vi "CODMn测量数据储存.vi"   [LabVIEW 2016, in "斯坦道CODMn新电路板.lvlib"]
uses:
  <vilib>/ptbypt/NI_PtbyPt.lvlib
types:
  T1 = cluster{"时间标识":timestamp, "监测值":sgl, "单位":u16, "数据标识":string, "因子编码":u32, "标样参考值":sgl, "A":sgl, "B":sgl, "K":sgl, "终点滴定数":sgl, "环境温度":sgl, "环境湿度":sgl, "量程":sgl, "加热实时温度":sgl, "X0":sgl, "X^2":sgl, "X":sgl, "B 2":sgl, "跨度值":sgl, "光值1":sgl, "光值2":sgl, "光值3":sgl, "光值4":sgl, "光值5":sgl, "光值6":sgl, "光值7":sgl, "光值8":sgl}
  T2 = enum16{"维护数据", "水样测试", "标样核查", "零点核查", "跨度核查", "空白测试", "平行样测试", "加标回收", "空白校准", "标样校准", "初始化（清洗）"}
  T3 = cluster{"系统时间":timestamp, "工作状态":u16, "测量模式":enum16{"待机", "连续模式", "周期模式", "定点模式", "受控模式", "手动模式"}, "告警代码":u16, "故障代码":u16, "日志代码":u16, "软件版本":u16, "A":sgl, "B":sgl, "K":sgl, "当前滴定数":sgl, "T":sgl, "H":sgl, "id":u16, "flowid":u16, "量程":u16, "加热实时温度":sgl, "当前ORP值":sgl, "运行时间":sgl, "当前步骤剩余时间":sgl, "结束滴定数":sgl, "注射泵保温温度":sgl, "匹配滴定数X0":u16, "X^2":sgl, "X":sgl, "B 2":sgl, "光值1":sgl, "光值2":sgl, "光值3":sgl, "光值4":sgl, "光值5":sgl, "光值6":sgl, "光值7":sgl, "光值8":sgl}
  T4 = enum16{"水样测试", "标样核查", "跨度核查", "零点核查", "空白测试", "平行样测试", "加标回收", "空白校准", "标样校准"}[]
  T5 = cluster{"运行模式":enum16{"维护模式", "常规模式", "应急模式", "质控模式", "性能测试"}, "质控频次":enum16{"关闭", "每天", "星期一", "星期二", "星期三", "星期四", "星期五", "星期六", "星期日"}, "空白核查时间":u16, "跨度核查时间":u16, "测量间隔":u16}
  T6 = cluster{"因子编码":u32, "单位":u16, "标样参考值":sgl, "水样数据时间":timestamp, "水样实测值":sgl, "水样数据标识":string, "标样数据时间":timestamp, "标样实测值":sgl, "标样数据标识":string, "空白数据时间":timestamp, "空白实测值":sgl, "空白数据标识":string, "零点核查数据时间":timestamp, "零点核查实测值":sgl, "零点核查数据标识":string, "跨度核查数据时间":timestamp, "跨度核查实测值":sgl, "跨度核查数据标识":string, "加标回收数据时间":timestamp, "加标回收实测值":sgl, "加标回收数据标识":string, "平行样数据时间":timestamp, "平行样实测值":sgl, "平行样数据标识":string, "F0":sgl, "F1":sgl, "F2":sgl, "F3":sgl, "F4":sgl, "F5":sgl, "F6":sgl, "F7":sgl, "温度":sgl, "湿度":sgl, "X值":sgl, "fidrange":u16}
  T7 = cluster{"跨度值":dbl, "零点标准液浓度":dbl, "跨度标准液浓度":dbl, "标准液标准浓度":dbl, "零点标准液偏差":dbl, "跨度标准液偏差":dbl, "标准液标准偏差":dbl}
  T8 = cluster{"公式":cluster{"X^2":dbl, "X":dbl, "B":dbl}, "校准":cluster{"校准？":bool, "校准点1-5":u16, "校准浓度":dbl}}
  T9 = cluster{"测量量程":sgl, "测量检出限":sgl, "测量精度":sgl, "测量间隔":sgl, "消解温度":sgl, "消解时长":sgl, "三项式系数":sgl, "二次多项式系数":sgl, "曲线斜率":sgl, "曲线截距":sgl, "线性相关系数":sgl, "空白校准时间":timestamp, "标样校准时间":timestamp, "测量信号值":sgl, "稀释倍数":sgl, "量程系数":sgl}
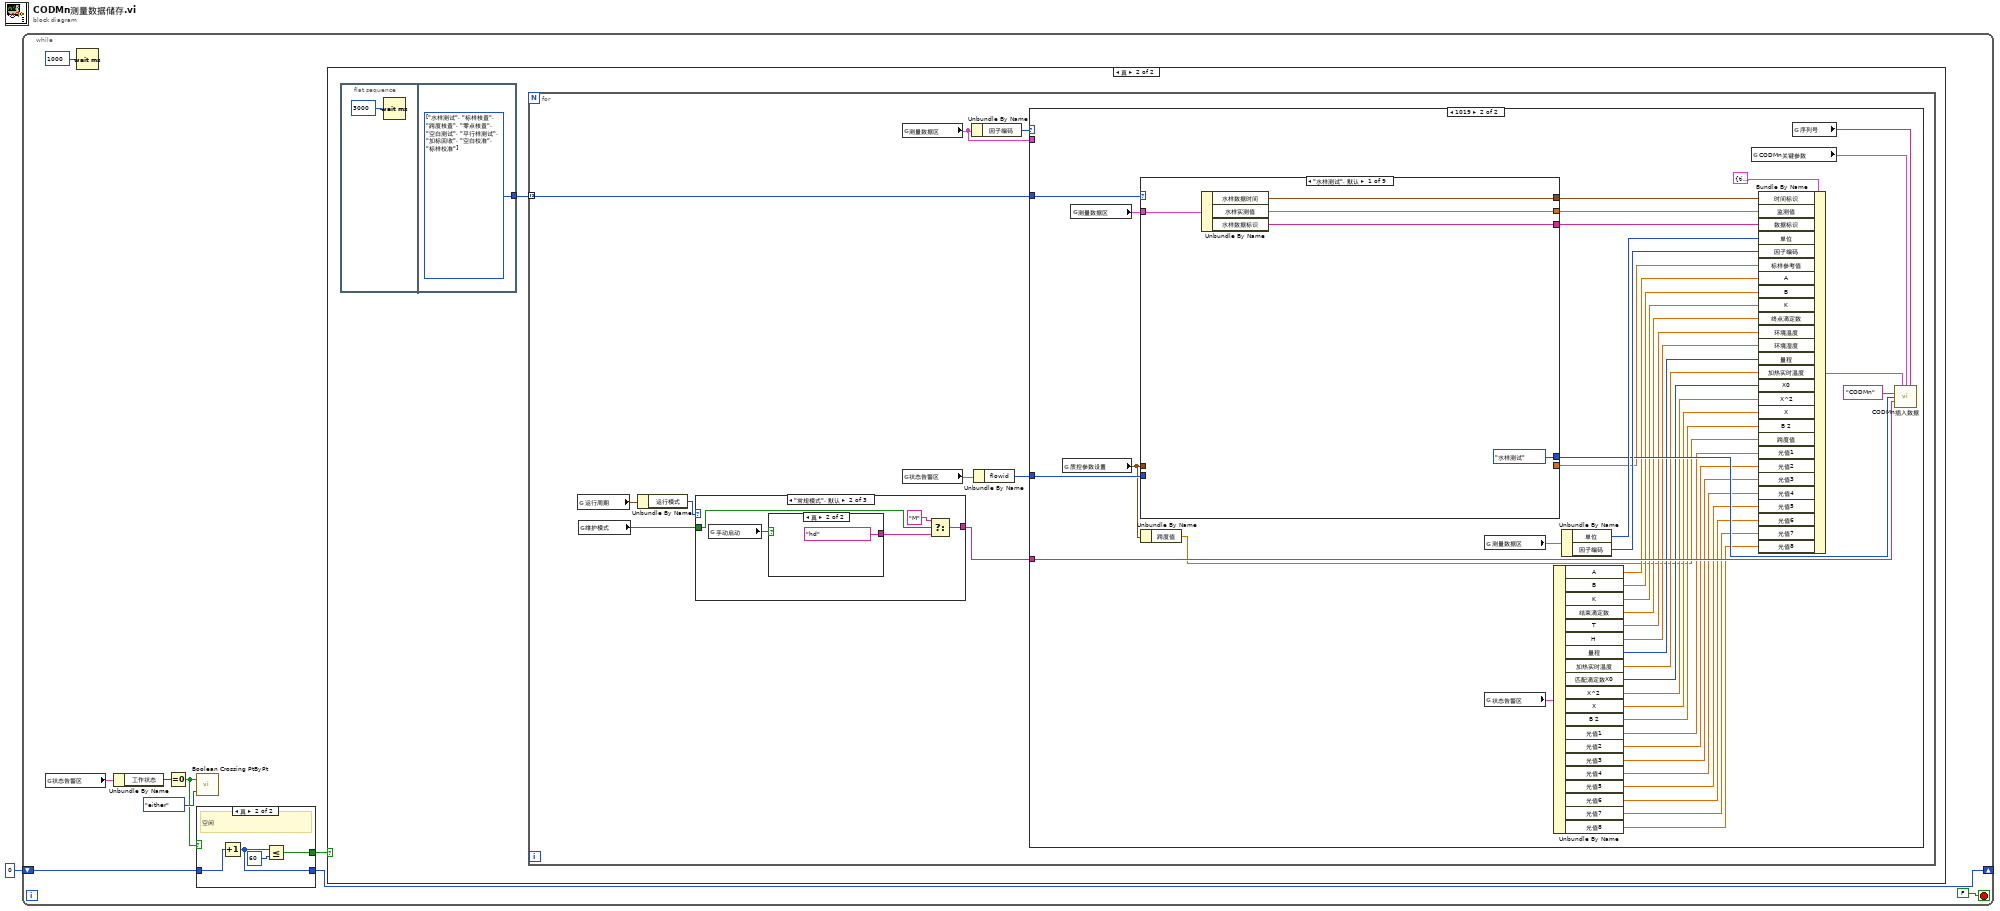
[diagram p0: block diagram]
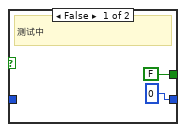
[diagram p2: hidden frame]
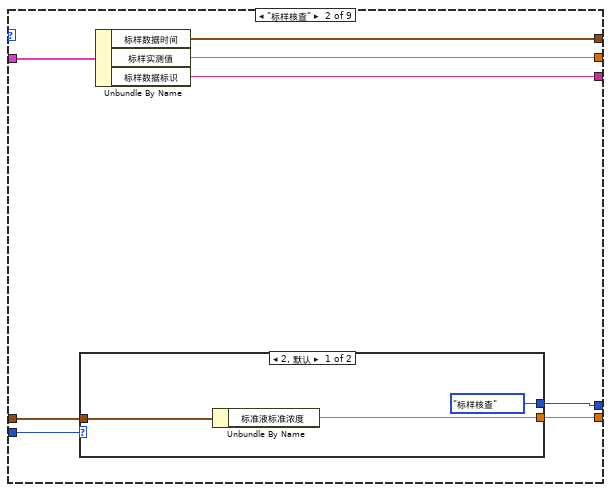
[diagram p5: hidden frame]
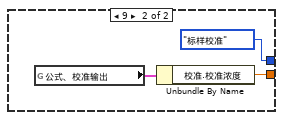
[diagram p6: hidden frame]
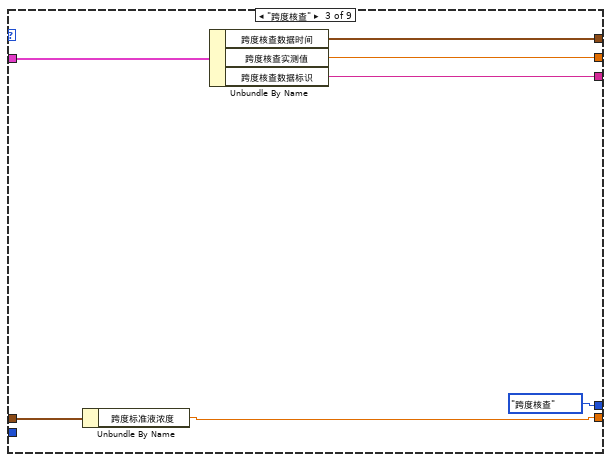
[diagram p7: hidden frame]
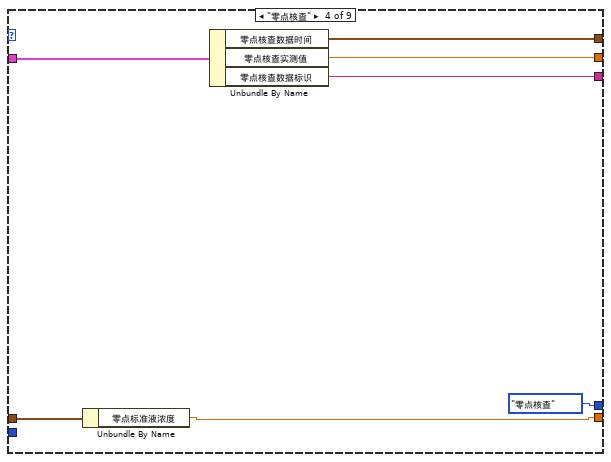
[diagram p8: hidden frame]
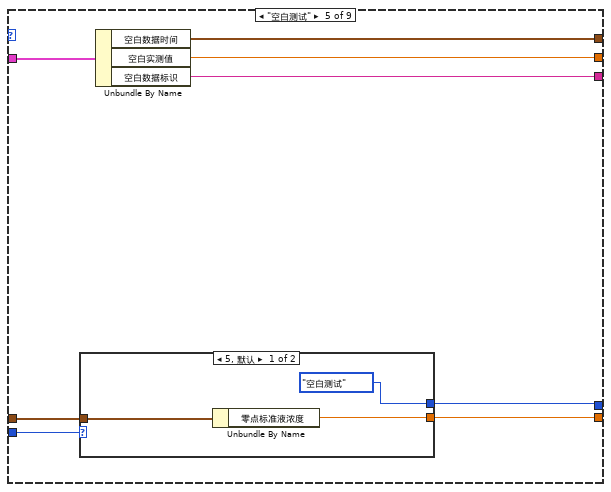
[diagram p9: hidden frame]
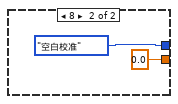
[diagram p10: hidden frame]
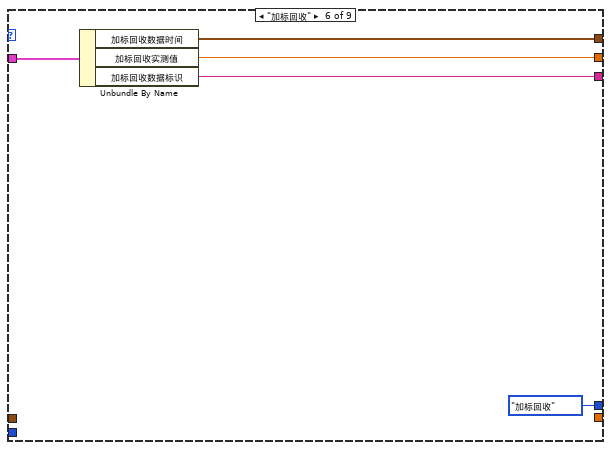
[diagram p11: hidden frame]
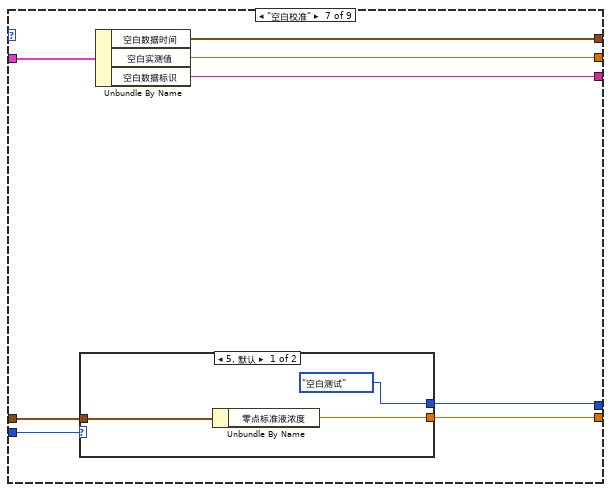
[diagram p12: hidden frame]
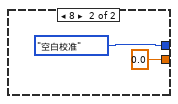
[diagram p13: hidden frame]
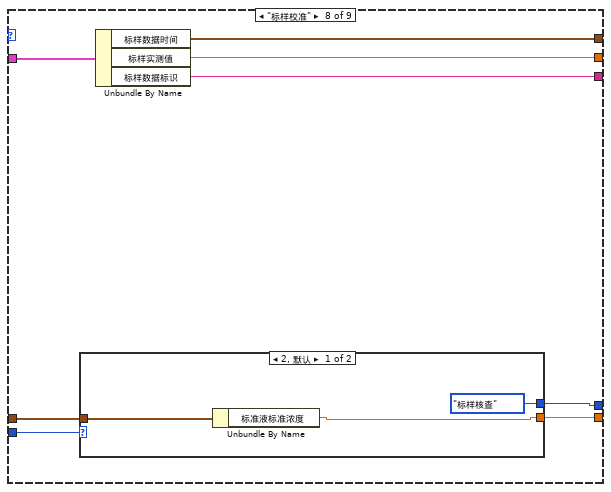
[diagram p14: hidden frame]
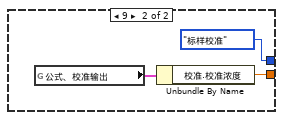
[diagram p15: hidden frame]
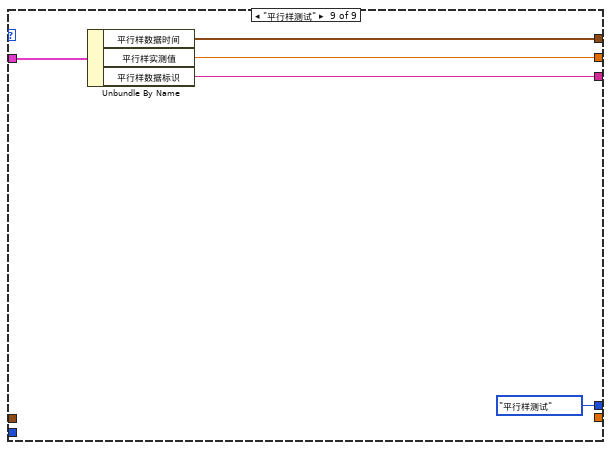
[diagram p16: hidden frame]
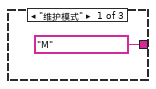
[diagram p17: hidden frame]
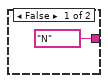
[diagram p18: hidden frame]
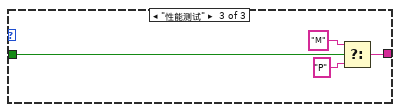
[diagram p19: hidden frame]
diagram:
  n1 = while {
    shift-right: [w3] -> _
    shift-left: 0 ("y") -> [w4]
    stop <- FALSE stop-if-true
    n2 = global read "VARCODMn全局变量.vi" "状态告警区"() -> (w7:T3)
    n3 = Wait (ms)(milliseconds to wait=u32 1000 ("等待时间（毫秒）")) -> ()  [unwired: 1 out]
    n4 = Unbundle By Name(w7) -> ("工作状态"=w6:u16)
    n5 = Equal To 0?(x=w6) -> (x = 0?=w5:bool)
    n6 = call <vilib>:"Boolean Crossing PtByPt.vi"("direction"=enum16{"either", "false-true", "true-false"}."either", "input"=w5) -> ()  [unwired: 1 in, 1 out]
    n7 = case shown="真" w5 {
      tunnel: w4 -> [_ w15]
      tunnel: [0 w14] -> w3
      tunnel: [FALSE w13] -> w2
      frame False {
        # "测试中"
      }
      frame True {
        # "空闲"
        n8 = Increment(x=w15) -> (x+1=w14:i32)
        n9 = Less Or Equal?(x=w14, y=u32 60) -> (x <= y?=w13:bool)
      }
    }
    n10 = case shown="真" w2 {
      frame False {
      }
      frame True {
        n11 = flat-sequence {
          tunnel: [w19] -> w17
          frame #0 {
            n12 = Wait (ms)(milliseconds to wait=u32 3000 ("等待时间（毫秒）")) -> ()  [unwired: 1 out]
          }
          frame #1 {
            w19 = T4 [enum."水样测试", enum."标样核查", enum."跨度核查", enum."零点核查", enum."空白测试", enum."平行样测试", enum."加标回收", enum."空白校准", enum."标样校准"] items=["水样测试", "标样核查", "跨度核查", "零点核查", "空白测试", "平行样测试", "加标回收", "空白校准", "标样校准"]
          }
        }
        n13 = for {
          tunnel: w17 -> [w27] mode=indexing
          n14 = global read "CODMn断电保存全局变量.vi" "运行周期"() -> (w24:T5)
          n15 = global read "VARCODMn全局变量.vi" "维护模式"() -> (w20:bool)
          n16 = Unbundle By Name(w24) -> ("运行模式"=w21:enum16{"维护模式", "常规模式", "应急模式", "质控模式", "性能测试"})
          n17 = case shown="\"常规模式\", 默认" w21 {
            tunnel: ["M" ("数据标记表") w153 w161] -> w28
            tunnel: w20 -> [_ w156 w163]
            frame "维护模式" {
            }
            frame "常规模式", Default {
              n18 = global read "VARCODMn全局变量.vi" "手动启动"() -> (w157:bool)
              n19 = case shown="真" w157 {
                tunnel: ["N" ("数据标记表") "hd" ("数据标记表")] -> w154
                frame False {
                }
                frame True {
                }
              }
              n20 = Select(t="M", s=w156, f=w154) -> (s? t:f=w153:string)
            }
            frame "性能测试" {
              n21 = Select(t="M", s=w163, f="P") -> (s? t:f=w161:string)
            }
          }
          n22 = global read "VARCODMn全局变量.vi" "测量数据区"() -> (w23:T6)
          n23 = global read "VARCODMn全局变量.vi" "状态告警区"() -> (w26:T3)
          n24 = Unbundle By Name(w23) -> ("因子编码"=w22:u32)
          n25 = Unbundle By Name(w26) -> ("flowid"=w25:u16)
          n26 = case shown="1019" w22 {
            tunnel: w23 -> [_ _]
            tunnel: w28 -> [_ w58]
            tunnel: w27 -> [_ w57]
            tunnel: w25 -> [_ w55]
            frame Default {
            }
            frame 1019 {
              n27 = global read "CODMn断电保存全局变量.vi" "质控参数设置"() -> (w40:T7)
              n28 = global read "VARCODMn全局变量.vi" "测量数据区"() -> (w68:T6)
              n29 = case shown="\"水样测试\", 默认" w57 {
                tunnel: w68 -> [w73 w81 w94 w101 w109 w119 w127 w140 w150]
                tunnel: [w72 w80 w93 w100 w108 w118 w126 w139 w149] -> w61
                tunnel: [w69 w79 w92 w99 w107 w115 w125 w138 w148] -> w62
                tunnel: [w71 w78 w91 w98 w106 w117 w124 w137 w147] -> w63
                tunnel: [T2."水样测试" ("测量模式") w76 T2."跨度核查" ("测量模式") T2."零点核查" ("测量模式") w104 T2."加标回收" ("测量模式") w121 w135 T2."平行样测试" ("测量模式")] -> w60
                tunnel: w40 -> [_ w74 w89 w96 w102 _ w120 w133 _]
                tunnel: [_ w75 w88 w95 w103 _ w123 w134 _] -> w56
                tunnel: w55 -> [_ w77 _ _ w105 _ w122 w136 _]
                frame "水样测试", Default {
                  n30 = Unbundle By Name(w73) -> ("水样数据时间"=w72:timestamp, "水样实测值"=w69:sgl, "水样数据标识"=w71:string)
                }
                frame "标样核查" {
                  n31 = case shown="2, 默认" w77 {
                    tunnel: [T2."标样核查" ("测量模式") T2."标样校准" ("测量模式")] -> w76
                    tunnel: [w82 w85] -> w75
                    tunnel: w74 -> [w83 _]
                    frame 2, Default {
                      n32 = Unbundle By Name(w83) -> ("标准液标准浓度"=w82:dbl)
                    }
                    frame 9 {
                      n33 = global read "CODMn断电保存全局变量.vi" "公式、校准输出"() -> (w86:T8)
                      n34 = Unbundle By Name(w86) -> ("校准.校准浓度"=w85:dbl)
                    }
                  }
                  n35 = Unbundle By Name(w81) -> ("标样数据时间"=w80:timestamp, "标样实测值"=w79:sgl, "标样数据标识"=w78:string)
                }
                frame "跨度核查" {
                  n36 = Unbundle By Name(w89) -> ("跨度标准液浓度"=w88:dbl)
                  n37 = Unbundle By Name(w94) -> ("跨度核查数据时间"=w93:timestamp, "跨度核查实测值"=w92:sgl, "跨度核查数据标识"=w91:string)
                }
                frame "零点核查" {
                  n38 = Unbundle By Name(w96) -> ("零点标准液浓度"=w95:dbl)
                  n39 = Unbundle By Name(w101) -> ("零点核查数据时间"=w100:timestamp, "零点核查实测值"=w99:sgl, "零点核查数据标识"=w98:string)
                }
                frame "空白测试" {
                  n40 = case shown="5, 默认" w105 {
                    tunnel: [T2."空白测试" ("测量模式") T2."空白校准" ("测量模式")] -> w104
                    tunnel: [w110 0.0 ("零点标准液浓度")] -> w103
                    tunnel: w102 -> [w111 _]
                    frame 5, Default {
                      n41 = Unbundle By Name(w111) -> ("零点标准液浓度"=w110:dbl)
                    }
                    frame 8 {
                    }
                  }
                  n42 = Unbundle By Name(w109) -> ("空白数据时间"=w108:timestamp, "空白实测值"=w107:sgl, "空白数据标识"=w106:string)
                }
                frame "加标回收" {
                  n43 = Unbundle By Name(w119) -> ("加标回收数据时间"=w118:timestamp, "加标回收实测值"=w115:sgl, "加标回收数据标识"=w117:string)
                }
                frame "空白校准" {
                  n44 = case shown="5, 默认" w122 {
                    tunnel: [T2."空白测试" ("测量模式") T2."空白校准" ("测量模式")] -> w121
                    tunnel: [w128 0.0 ("零点标准液浓度")] -> w123
                    tunnel: w120 -> [w129 _]
                    frame 5, Default {
                      n45 = Unbundle By Name(w129) -> ("零点标准液浓度"=w128:dbl)
                    }
                    frame 8 {
                    }
                  }
                  n46 = Unbundle By Name(w127) -> ("空白数据时间"=w126:timestamp, "空白实测值"=w125:sgl, "空白数据标识"=w124:string)
                }
                frame "标样校准" {
                  n47 = case shown="2, 默认" w136 {
                    tunnel: [T2."标样核查" ("测量模式") T2."标样校准" ("测量模式")] -> w135
                    tunnel: [w141 w144] -> w134
                    tunnel: w133 -> [w142 _]
                    frame 2, Default {
                      n48 = Unbundle By Name(w142) -> ("标准液标准浓度"=w141:dbl)
                    }
                    frame 9 {
                      n49 = global read "CODMn断电保存全局变量.vi" "公式、校准输出"() -> (w145:T8)
                      n50 = Unbundle By Name(w145) -> ("校准.校准浓度"=w144:dbl)
                    }
                  }
                  n51 = Unbundle By Name(w140) -> ("标样数据时间"=w139:timestamp, "标样实测值"=w138:sgl, "标样数据标识"=w137:string)
                }
                frame "平行样测试" {
                  n52 = Unbundle By Name(w150) -> ("平行样数据时间"=w149:timestamp, "平行样实测值"=w148:sgl, "平行样数据标识"=w147:string)
                }
              }
              n53 = Unbundle By Name(w40) -> ("跨度值"=w39:dbl)
              n54 = global read "VARCODMn全局变量.vi" "测量数据区"() -> (w65:T6)
              n55 = global read "VARCODMn全局变量.vi" "状态告警区"() -> (w54:T3)
              n56 = Unbundle By Name(w54) -> ("A"=w47:sgl, "B"=w53:sgl, "K"=w48:sgl, "结束滴定数"=w49:sgl, "T"=w50:sgl, "H"=w46:sgl, "量程"=w51:u16, "加热实时温度"=w52:sgl, "匹配滴定数X0"=w45:u16, "X^2"=w42:sgl, "X"=w43:sgl, "B 2"=w44:sgl, "光值1"=w37:sgl, "光值2"=w36:sgl, "光值3"=w35:sgl, "光值4"=w34:sgl, "光值5"=w33:sgl, "光值6"=w32:sgl, "光值7"=w31:sgl, "光值8"=w30:sgl)
              n57 = Unbundle By Name(w65) -> ("单位"=w67:u16, "因子编码"=w66:u32)
              n58 = global read "CODMn断电保存全局变量.vi" "CODMn关键参数"() -> (w41:T9)
              n59 = Bundle By Name(cluster=T1 {"时间标识"=timestamp(0 s since 1904-01-01), "监测值"=0.0, "单位"=0, "数据标识"="", "因子编码"=0, "标样参考值"=0.0, "A"=0.0, "B"=0.0, "K"=0.0, "终点滴定数"=0.0, "环境温度"=0.0, "环境湿度"=0.0, "量程"=0.0, "加热实时温度"=0.0, "X0"=0.0, "X^2"=0.0, "X"=0.0, "B 2"=0.0, "跨度值"=0.0, "光值1"=0.0, "光值2"=0.0, "光值3"=0.0, "光值4"=0.0, "光值5"=0.0, "光值6"=0.0, "光值7"=0.0, "光值8"=0.0} ("data"), "时间标识"=w61, "监测值"=w62, "数据标识"=w63, "单位"=w67, "因子编码"=w66, "标样参考值"=w56, "A"=w47, "B"=w53, "K"=w48, "终点滴定数"=w49, "环境温度"=w50, "环境湿度"=w46, "量程"=w51, "加热实时温度"=w52, "X0"=w45, "X^2"=w42, "X"=w43, "B 2"=w44, "跨度值"=w39, "光值1"=w37, "光值2"=w36, "光值3"=w35, "光值4"=w34, "光值5"=w33, "光值6"=w32, "光值7"=w31, "光值8"=w30) -> (w29:T1)
              n60 = global read "VARCODMn全局变量.vi" "序列号"() -> (w64:string)
              n61 = call "CODMn插入数据.vi"("data"=w29, "CODMn关键参数"=w41, "SN"=w64, "table"="CODMn", "测量模式"=w60, "数据类型"=w58) -> ()  [unwired: 9 in, 1 out]
            }
          }
        }
      }
    }
  }
